vi "OverlyLocations.vi"(8 "error in (no error)":errorcluster, 10 "FaceLocations":refnum<k24>, 11 "Image in":T1) -> (0 "error out":errorcluster, 2 "FaceLocations out":refnum<k24>, 3 "Image Out":T1)   [LabVIEW 2020]
uses:
  <vilib>/vision/Image Controls.llb/IMAQ Image.ctl
  FaceRecognition.lvclass
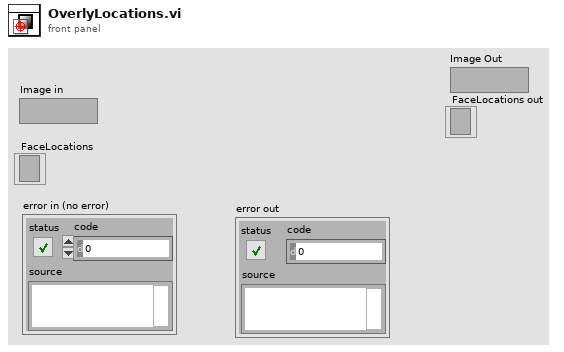
[diagram p1: front panel]
types:
  T1 = typedef "IMAQ Image.ctl" = refnum<image>
  T2 = typedef "FaceRecognitionDotNet.lvlib/FaceRecognition.lvclass/Location.ctl" = cluster{"Left":i32, "Top":i32, "Right":i32, "Bottom":i32}
  T3 = cluster{"Desired Font (Application)":enum16{"User-specified Font", "Application Font", "System Font", "Dialog Font"}, "[User-specified Font]":cluster{"Font Name":string, "Size":i16, "Strikeout?":bool, "Italic?":bool, "Underline?":bool, "Outline?":bool, "Shadow?":bool, "Bold?":bool, "Rotation Angle":dbl}, "Horizontal Alignment":i16, "Vertical Alignment":i16}
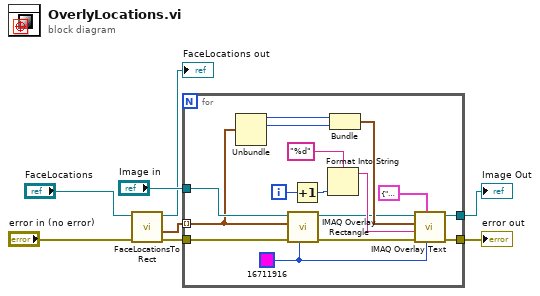
[diagram p0: block diagram]
diagram:
  n1 = call "FaceLocationsToRect.vi"("error in (no error)"="error in (no error)", "FaceLocations"="FaceLocations") -> ("error out"=w3:errorcluster, "Locations"=w7:T2[], "FaceLocations out"=→"FaceLocations out":refnum<k24>)  [unwired: 7 in]
  n2 = for {
    tunnel: w7 -> [w16] mode=indexing
    tunnel: "Image in" -> [w18]
    tunnel: w3 -> [w17]
    tunnel: [w10] -> w5
    tunnel: [w9] -> w6
    i -> [w24]
    w20 = u32 16711916 ("Color")
    n3 = Unbundle(w16) -> ("Left"=w15:i32, "Top"=w14:i32)  [unwired: 2 out]
    n4 = call "IMAQ Overlay Rectangle"("Color"=w20, "error in (no error)"=w17, "Rectangle"=w16, "Image"=w18) -> ("error out"=w11:errorcluster, "Image Out"=w12:T1)  [unwired: 6 in]
    n5 = Increment(x=w24) -> (x+1=w23:i32)
    n6 = Format Into String(format string="%d", w23) -> (resulting string=w21:string)  [unwired: 2 in, 1 out]
    n7 = Bundle("Left"=w15, "Top"=w14) -> (w13:cluster{"Left":i32, "Top":i32})  [unwired: 1 in]
    n8 = call "IMAQ Overlay Text"("Text Color (black)"=w20, "Font, Size & Style"=T3 {"Desired Font (Application)"=enum."System Font", "[User-specified Font]"={"Font Name"="Tahoma", "Size"=100, "Strikeout?"=FALSE, "Italic?"=FALSE, "Underline?"=FALSE, "Outline?"=FALSE, "Shadow?"=FALSE, "Bold?"=FALSE, "Rotation Angle"=0.0}, "Horizontal Alignment"=0, "Vertical Alignment"=0}, "error in (no error)"=w11, "String"=w21, "Origin"=w13, "Image"=w12) -> ("error out"=w9:errorcluster, "Image Out"=w10:T1)  [unwired: 4 in]
  }
  "error out" <- w6
  "Image Out" <- w5
